vi "rowcol2xlscell.vi"(2 "XLS column":u32, 3 "XLS row":u32) -> (0 "column":string, 1 "XLS cell":string)   [LabVIEW 2013]
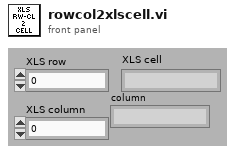
[diagram p1: front panel]
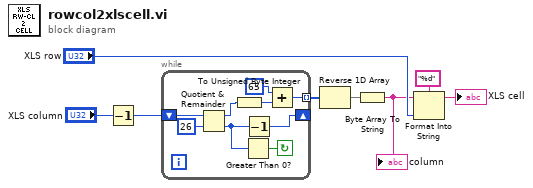
[diagram p0: block diagram]
diagram:
  n1 = Decrement(x="XLS column") -> (x-1=w1:u32)
  n2 = while {
    shift-right: [w9] -> _
    shift-left: w1 -> [w17]
    tunnel: [w12] -> w5 mode=indexing
    stop <- w13 continue-if-true
    n3 = Quotient & Remainder(x=w17, y=u32 26) -> (x-y*floor(x/y)=w15:u32, floor(x/y)=w11:u32)
    n4 = To Unsigned Byte Integer(number=w15) -> (unsigned 8bit integer=w10:u8)
    n5 = Greater Than 0?(x=w11) -> (x > 0?=w13:bool)
    n6 = Decrement(x=w11) -> (x-1=w9:u32)
    n7 = Add(x=u8 65, y=w10) -> (x+y=w12:u8)
  }
  n8 = Reverse 1D Array(array=w5) -> (reversed array=w4:u8[])
  n9 = Byte Array To String(unsigned byte array=w4) -> (string=w3:string)
  "column" <- w3
  n10 = Format Into String(format string="%d", initial string=w3, "XLS row") -> (resulting string=→"XLS cell":string)  [unwired: 1 in, 1 out]
